vi "Supported Smart Syntax Representation.vi"(0 "Message Popup in":refnum<class "UI Functions.lvclass">, 11 "error in (no error)":errorcluster) -> (4 "Message Popup out":refnum<class "UI Functions.lvclass">, 6 "Smart Syntax Representation List":string[](array[string]), 15 "error out":errorcluster)   [LabVIEW 2019, in "UI Functions.lvclass"]
uses:
  UI Functions.lvclass
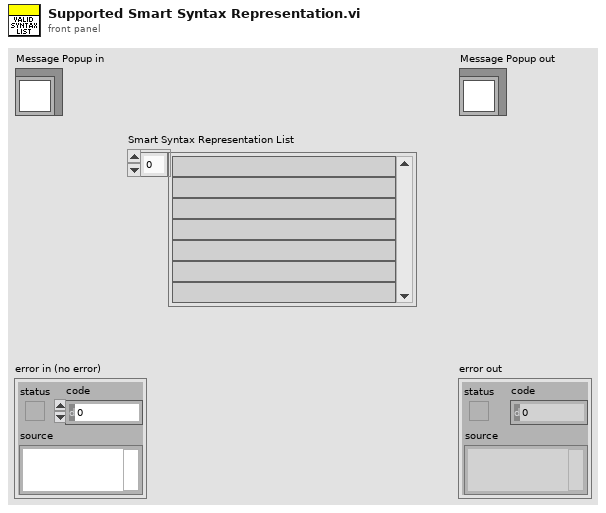
[diagram p1: front panel]
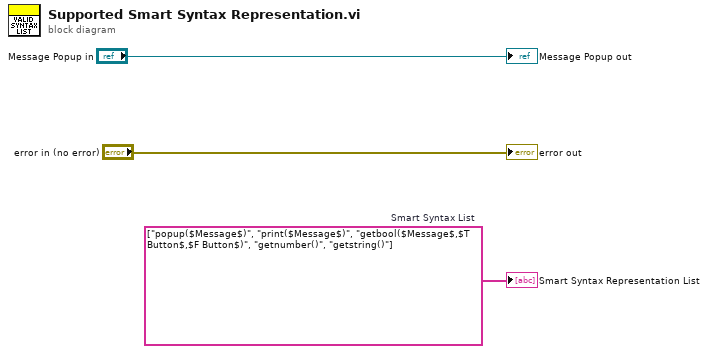
[diagram p0: block diagram]
diagram:
  w1 = string[] ["popup($Message$)", "print($Message$)", "getbool($Message$,$T Button$,$F Button$)", "getnumber()", "getstring()"]  # Smart Syntax List
  "error out" <- "error in (no error)"
  "Message Popup out" <- "Message Popup in"
  "Smart Syntax Representation List" <- w1
